vi "DisplayJson.vi"(11 "JSON String In":string="[{\"version\":\"1.0.0\",\"header\":{\"creationDate\":\"2022-06-03T00:00:00\",\"remarks\":\"\",\"serialNumber\":\"98172\",\"productNumber\":\"123021.1804\",\"productType\":\"PAA-9L\",\"pressureType\":2,\"productSeries\":\"9L\",\"compensatedTemperatureRange\":{\"min\":-10.0,\"max\":80.0,\"unit\":4},\"compensatedPressureRange\":{\"min\":0.0,\"max\":0.35,\"unit\":3},\"electricSupply\":{\"magnitude\":1.0,\"unit\":18},\"orderNumber\":9990266,\"orderPosition\":3,\"orderTargetDispatchDate\":\"2022-06-02T00:00:00+00:00\",\"customerName\":\"DemoData Inc.\",\"customerNumber\":12345678,\"customerOrderNumber\":\"Cust-9990266-123\",\"customerReferenceNumber\":\"\",\"customerProductT...") -> ()   [LabVIEW 2017] (continued)
nsatedPressureRange\":{\"min\":0.0,\"max\":0.35,\"unit\":3},\"electricSupply\":{\"magnitude\":1.0,\"unit\":18},\"parts\":{\"pressure\":{\"inputs\":[\"Sig\",\"R\"],\"output\":\"P\",\"description\":\"P = f(Sig,R)\",\"coefficients\":[[4.32580143572,-0.00440494166515,1.6640292116E-06,-2.811503068E-10,1.77714318789E-14],[-0.135698051026,0.000145399145759,-5.51829171562E-08,9.2954527005E-12,-5.87658681908E-16],[-0.000210397340774,2.63566870768E-07,-1.19781998432E-10,2.37289366107E-14,-1.74028064372E-18]]},\"temperature\":{\"inputs\":[\"R\",\"Sig\"],\"output\":\"T\",\"description\":\"T = f(R,Sig)\",\"coefficients\":[[-7912.16489659,3.11303262224,-0.10735561471],[7.82433050485,-0.00250618716574,0.000118515503682],[-0.00296929079857,7.28944709623E-07,-4.91144781497E-08],[5.10659036054E-07,-8.59548259995E-11,9.04763177647E-12],[-3.31476837963E-11,3.07780227507E-15,-6.24752257771E-16]]}}}}},\"measurements\":[{\"reference\":\"F_12300_XX_0000098765\",\"environmentTarget\":{\"pressure\":{\"magnitude\":0.03,\"unit\":3},\"temperature\":{\"magnitude\":-10.0,\"unit\":4}},\"environment\":{\"pressure\":{\"magnitude\":0.030005,\"unit\":3},\"temperature\":{\"magnitude\":-10.7286,\"unit\":4},\"supply\":{\"magnitude\":1.0,\"unit\":18}},\"raw\":{\"signal\":{\"magnitude\":15.068338109,\"unit\":22},\"bridgeResistance\":{\"magnitude\":3268.0076497,\"unit\":28}},\"compensated\":{\"mathematicalModels\":{\"MM0123\":{\"pressure\":{\"output\":{\"magnitude\":0.0300137,\"unit\":3},\"error\":{\"magnitude\":0.0024720218,\"unit\":7}},\"temperature\":{\"output\":{\"magnitude\":-10.8267,\"unit\":4},\"error\":{\"magnitude\":-0.098057362,\"unit\":4}}}}}},{\"reference\":\"F_12300_XX_0000098765\",\"environmentTarget\":{\"pressure\":{\"magnitude\":0.11,\"unit\":3},\"temperature\":{\"magnitude\":-10.0,\"unit\":4}},\"environment\":{\"pressure\":{\"magnitude\":0.109989,\"unit\":3},\"temperature\":{\"magnitude\":-10.7286,\"unit\":4},\"supply\":{\"magnitude\":1.0,\"unit\":18}},\"raw\":{\"signal\":{\"magnitude\":25.595891825,\"unit\":22},\"bridgeResistance\":{\"magnitude\":3264.0622557,\"unit\":28}},\"compensated\":{\"mathematicalModels\":{\"MM0123\":{\"pressure\":{\"output\":{\"magnitude\":0.10996,\"unit\":3},\"error\":{\"magnitude\":-0.0079711693,\"unit\":7}},\"temperature\":{\"output\":{\"magnitude\":-10.8338,\"unit\":4},\"error\":{\"magnitude\":-0.10516508,\"unit\":4}}}}}},{\"reference\":\"F_12300_XX_0000098765\",\"environmentTarget\":{\"pressure\":{\"magnitude\":0.19,\"unit\":3},\"temperature\":{\"magnitude\":-10.0,\"unit\":4}},\"environment\":{\"pressure\":{\"magnitude\":0.190009,\"unit\":3},\"temperature\":{\"magnitude\":-10.7286,\"unit\":4},\"supply\":{\"magnitude\":1.0,\"unit\":18}},\"raw\":{\"signal\":{\"magnitude\":36.103007271,\"unit\":22},\"bridgeResistance\":{\"magnitude\":3260.2938754,\"unit\":28}},\"compensated\":{\"mathematicalModels\":{\"MM0123\":{\"pressure\":{\"output\":{\"magnitude\":0.190015,\"unit\":3},\"error\":{\"magnitude\":0.001783636,\"unit\":7}},\"temperature\":{\"output\":{\"magnitude\":-10.8272,\"unit\":4},\"error\":{\"magnitude\":-0.098521286,\"unit\":4}}}}}},{\"reference\":\"F_12300_XX_0000098765\",\"environmentTarget\":{\"pressure\":{\"magnitude\":0.27,\"unit\":3},\"temperature\":{\"magnitude\":-10.0,\"unit\":4}},\"environment\":{\"pressure\":{\"magnitude\":0.270007,\"unit\":3},\"temperature\":{\"magnitude\":-10.7286,\"unit\":4},\"supply\":{\"magnitude\":1.0,\"unit\":18}},\"raw\":{\"signal\":{\"magnitude\":46.569581681,\"unit\":22},\"bridgeResistance\":{\"magnitude\":3256.5849623,\"unit\":28}},\"compensated\":{\"mathematicalModels\":{\"MM0123\":{\"pressure\":{\"output\":{\"magnitude\":0.270034,\"unit\":3},\"error\":{\"magnitude\":0.0075826501,\"unit\":7}},\"temperature\":{\"output\":{\"magnitude\":-10.8257,\"unit\":4},\"error\":{\"magnitude\":-0.097105964,\"unit\":4}}}}}},{\"reference\":\"F_12300_XX_0000098765\",\"environmentTarget\":{\"pressure\":{\"magnitude\":0.35,\"unit\":3},\"temperature\":{\"magnitude\":-10.0,\"unit\":4}},\"environment\":{\"pressure\":{\"magnitude\":0.350004,\"unit\":3},\"temperature\":{\"magnitude\":-10.7286,\"unit\":4},\"supply\":{\"magnitude\":1.0,\"unit\":18}},\"raw\":{\"signal\":{\"magnitude\":56.993492418,\"unit\":22},\"bridgeResistance\":{\"magnitude\":3252.9352126,\"unit\":28}},\"compensated\":{\"mathematicalModels\":{\"MM0123\":{\"pressure\":{\"output\":{\"magnitude\":0.35,\"unit\":3},\"error\":{\"magnitude\":-0.0012287617,\"unit\":7}},\"temperature\":{\"output\":{\"magnitude\":-10.83,\"unit\":4},\"error\":{\"magnitude\":-0.10133045,\"unit\":4}}}}}},{\"reference\":\"F_12300_XX_0000098765\",\"environmentTarget\":{\"pressure\":{\"magnitude\":0.03,\"unit\":3},\"temperature\":{\"magnitude\":0.0,\"unit\":4}},\"environment\":{\"pressure\":{\"magnitude\":0.0299941,\"unit\":3},\"temperature\":{\"magnitude\":-0.629962,\"unit\":4},\"supply\":{\"magnitude\":1.0,\"unit\":18}},\"raw\":{\"signal\":{\"magnitude\":15.503162041,\"unit\":22},\"bridgeResistance\":{\"magnitude\":3337.8630039,\"unit\":28}},\"compensated\":{\"mathematicalModels\":{\"MM0123\":{\"pressure\":{\"output\":{\"magnitude\":0.0300113,\"unit\":3},\"error\":{\"magnitude\":0.0049240687,\"unit\":7}},\"temperature\":{\"output\":{\"magnitude\":-0.740587,\"unit\":4},\"error\":{\"magnitude\":-0.1106252,\"unit\":4}}}}}},{\"reference\":\"F_12300_XX_0000098765\",\"environmentTarget\":{\"pressure\":{\"magnitude\":0.11,\"unit\":3},\"temperature\":{\"magnitude\":0.0,\"unit\":4}},\"environment\":{\"pressure\":{\"magnitude\":0.110002,\"unit\":3},\"temperature\":{\"magnitude\":-0.629962,\"unit\":4},\"supply\":{\"magnitude\":1.0,\"unit\":18}},\"raw\":{\"signal\":{\"magnitude\":26.002306136,\"unit\":22},\"bridgeResistance\":{\"magnitude\":3333.9686869,\"unit\":28}},\"compensated\":{\"mathematicalModels\":{\"MM0123\":{\"pressure\":{\"output\":{\"magnitude\":0.10998,\"unit\":3},\"error\":{\"magnitude\":-0.0063838503,\"unit\":7}},\"temperature\":{\"output\":{\"magnitude\":-0.740425,\"unit\":4},\"error\":{\"magnitude\":-0.11046359,\"unit\":4}}}}}},{\"reference\":\"F_12300_XX_0000098765\",\"environmentTarget\":{\"pressure\":{\"magnitude\":0.19,\"unit\":3},\"temperature\":{\"magnitude\":0.0,\"unit\":4}},\"environment\":{\"pressure\":{\"magnitude\":0.190006,\"unit\":3},\"temperature\":{\"magnitude\":-0.629962,\"unit\":4},\"supply\":{\"magnitude\":1.0,\"unit\":18}},\"raw\":{\"signal\":{\"magnitude\":36.476080101,\"unit\":22},\"bridgeResistance\":{\"magnitude\":3330.1476544,\"unit\":28}},\"compensated\":{\"mathematicalModels\":{\"MM0123\":{\"pressure\":{\"output\":{\"magnitude\":0.190009,\"unit\":3},\"error\":{\"magnitude\":0.0007371048,\"unit\":7}},\"temperature\":{\"output\":{\"magnitude\":-0.741023,\"unit\":4},\"error\":{\"magnitude\":-0.11206099,\"unit\":4}}}}}},{\"reference\":\"F_12300_XX_0000098765\",\"environmentTarget\":{\"pressure\":{\"magnitude\":0.27,\"unit\":3},\"temperature\":{\"magnitude\":0.0,\"unit\":4}},\"environment\":{\"pressure\":{\"magnitude\":0.269998,\"unit\":3},\"temperature\":{\"magnitude\":-0.629962,\"unit\":4},\"supply\":{\"magnitude\":1.0,\"unit\":18}},\"raw\":{\"signal\":{\"magnitude\":46.912344811,\"unit\":22},\"bridgeResistance\":{\"magnitude\":3326.3598207,\"unit\":28}},\"compensated\":{\"mathematicalModels\":{\"MM0123\":{\"pressure\":{\"output\":{\"magnitude\":0.270009,\"unit\":3},\"error\":{\"magnitude\":0.0030303754,\"unit\":7}},\"temperature\":{\"output\":{\"magnitude\":-0.748735,\"unit\":4},\"error\":{\"magnitude\":-0.11877286,\"unit\":4}}}}}},{\"reference\":\"F_12300_XX_0000098765\",\"environmentTarget\":{\"pressure\":{\"magnitude\":0.35,\"unit\":3},\"temperature\":{\"magnitude\":0.0,\"unit\":4}},\"environment\":{\"pressure\":{\"magnitude\":0.350003,\"unit\":3},\"temperature\":{\"magnitude\":-0.629962,\"unit\":4},\"supply\":{\"magnitude\":1.0,\"unit\":18}},\"raw\":{\"signal\":{\"magnitude\":57.311280041,\"unit\":22},\"bridgeResistance\":{\"magnitude\":3322.6985202,\"unit\":28}},\"compensated\":{\"mathematicalModels\":{\"MM0123\":{\"pressure\":{\"output\":{\"magnitude\":0.349978,\"unit\":3},\"error\":{\"magnitude\":-0.007067618,\"unit\":7}},\"temperature\":{\"output\":{\"magnitude\":-0.750753,\"unit\":4},\"error\":{\"magnitude\":-0.12079072,\"unit\":4}}}}}},{\"reference\":\"F_12300_XX_0000098765\",\"environmentTarget\":{\"pressure\":{\"magnitude\":0.03,\"unit\":3},\"temperature\":{\"magnitude\":20.0,\"unit\":4}},\"environment\":{\"pressure\":{\"magnitude\":0.0299999,\"unit\":3},\"temperature\":{\"magnitude\":19.5509,\"unit\":4},\"supply\":{\"magnitude\":1.0,\"unit\":18}},\"raw\":{\"signal\":{\"magnitude\":16.409278781,\"unit\":22},\"bridgeResistance\":{\"magnitude\":3494.5350045,\"unit\":28}},\"compensated\":{\"mathematicalModels\":{\"MM0123\":{\"pressure\":{\"output\":{\"magnitude\":0.0300059,\"unit\":3},\"error\":{\"magnitude\":0.0017026825,\"unit\":7}},\"temperature\":{\"output\":{\"magnitude\":19.5499,\"unit\":4},\"error\":{\"magnitude\":-0.0009297112,\"unit\":4}}}}}},{\"reference\":\"F_12300_XX_0000098765\",\"environmentTarget\":{\"pressure\":{\"magnitude\":0.11,\"unit\":3},\"temperature\":{\"magnitude\":20.0,\"unit\":4}},\"environment\":{\"pressure\":{\"magnitude\":0.109998,\"unit\":3},\"temperature\":{\"magnitude\":19.5509,\"unit\":4},\"supply\":{\"magnitude\":1.0,\"unit\":18}},\"raw\":{\"signal\":{\"magnitude\":26.89717523,\"unit\":22},\"bridgeResistance\":{\"magnitude\":3490.6076187,\"unit\":28}},\"compensated\":{\"mathematicalModels\":{\"MM0123\":{\"pressure\":{\"output\":{\"magnitude\":0.109972,\"unit\":3},\"error\":{\"magnitude\":-0.0073489568,\"unit\":7}},\"temperature\":{\"output\":{\"magnitude\":19.5448,\"unit\":4},\"error\":{\"magnitude\":-0.0060927679,\"unit\":4}}}}}},{\"reference\":\"F_12300_XX_0000098765\",\"environmentTarget\":{\"pressure\":{\"magnitude\":0.19,\"unit\":3},\"temperature\":{\"magnitude\":20.0,\"unit\":4}},\"environment\":{\"pressure\":{\"magnitude\":0.189997,\"unit\":3},\"temperature\":{\"magnitude\":19.5509,\"unit\":4},\"supply\":{\"magnitude\":1.0,\"unit\":18}},\"raw\":{\"signal\":{\"magnitude\":37.363996162,\"unit\":22},\"bridgeResistance\":{\"magnitude\":3486.7813876,\"unit\":28}},\"compensated\":{\"mathematicalModels\":{\"MM0123\":{\"pressure\":{\"output\":{\"magnitude\":0.190001,\"unit\":3},\"error\":{\"magnitude\":0.0011381596,\"unit\":7}},\"temperature\":{\"output\":{\"magnitude\":19.5437,\"unit\":4},\"error\":{\"magnitude\":-0.0071879925,\"unit\":4}}}}}},{\"reference\":\"F_12300_XX_0000098765\",\"environmentTarget\":{\"pressure\":{\"magnitude\":0.27,\"unit\":3},\"temperature\":{\"magnitude\":20.0,\"unit\":4}},\"environment\":{\"pressure\":{\"magnitude\":0.269992,\"unit\":3},\"temperature\":{\"magnitude\":19.5509,\"unit\":4},\"supply\":{\"magnitude\":1.0,\"unit\":18}},\"raw\":{\"signal\":{\"magnitude\":47.800155632,\"unit\":22},\"bridgeResistance\":{\"magnitude\":3483.0010425,\"unit\":28}},\"compensated\":{\"mathematicalModels\":{\"MM0123\":{\"pressure\":{\"output\":{\"magnitude\":0.270022,\"unit\":3},\"error\":{\"magnitude\":0.008607717,\"unit\":7}},\"temperature\":{\"output\":{\"magnitude\":19.5395,\"unit\":4},\"error\":{\"magnitude\":-0.011423775,\"unit\":4}}}}}},{\"reference\":\"F_12300_XX_0000098765\",\"environmentTarget\":{\"pressure\":{\"magnitude\":0.35,\"unit\":3},\"temperature\":{\"magnitude\":20.0,\"unit\":4}},\"environment\":{\"pressure\":{\"magnitude\":0.350005,\"unit\":3},\"temperature\":{\"magnitude\":19.5509,\"unit\":4},\"supply\":{\"magnitude\":1.0,\"unit\":18}},\"raw\":{\"signal\":{\"magnitude\":58.202570119,\"unit\":22},\"bridgeResistance\":{\"magnitude\":3479.3453591,\"unit\":28}},\"compensated\":{\"mathematicalModels\":{\"MM0123\":{\"pressure\":{\"output\":{\"magnitude\":0.350009,\"unit\":3},\"error\":{\"magnitude\":0.0010923873,\"unit\":7}},\"temperature\":{\"output\":{\"magnitude\":19.5414,\"unit\":4},\"error\":{\"magnitude\":-0.009468969,\"unit\":4}}}}}},{\"reference\":\"F_12300_XX_0000098765\",\"environmentTarget\":{\"pressure\":{\"magnitude\":0.03,\"unit\":3},\"temperature\":{\"magnitude\":40.0,\"unit\":4}},\"environment\":{\"pressure\":{\"magnitude\":0.0299981,\"unit\":3},\"temperature\":{\"magnitude\":39.7284,\"unit\":4},\"supply\":{\"magnitude\":1.0,\"unit\":18}},\"raw\":{\"signal\":{\"magnitude\":17.383077086,\"unit\":22},\"bridgeResistance\":{\"magnitude\":3670.0301141,\"unit\":28}},\"compensated\":{\"mathematicalModels\":{\"MM0123\":{\"pressure\":{\"output\":{\"magnitude\":0.0300152,\"unit\":3},\"error\":{\"magnitude\":0.0048902957,\"unit\":7}},\"temperature\":{\"output\":{\"magnitude\":39.719,\"unit\":4},\"error\":{\"magnitude\":-0.0094604345,\"unit\":4}}}}}},{\"reference\":\"F_12300_XX_0000098765\",\"environmentTarget\":{\"pressure\":{\"magnitude\":0.11,\"unit\":3},\"temperature\":{\"magnitude\":40.0,\"unit\":4}},\"environment\":{\"pressure\":{\"magnitude\":0.109992,\"unit\":3},\"temperature\":{\"magnitude\":39.7284,\"unit\":4},\"supply\":{\"magnitude\":1.0,\"unit\":18}},\"raw\":{\"signal\":{\"magnitude\":27.915913124,\"unit\":22},\"bridgeResistance\":{\"magnitude\":3666.1287959,\"unit\":28}},\"compensated\":{\"mathematicalModels\":{\"MM0123\":{\"pressure\":{\"output\":{\"magnitude\":0.109964,\"unit\":3},\"error\":{\"magnitude\":-0.0079924079,\"unit\":7}},\"temperature\":{\"output\":{\"magnitude\":39.718,\"unit\":4},\"error\":{\"magnitude\":-0.010393948,\"unit\":4}}}}}},{\"reference\":\"F_12300_XX_0000098765\",\"environmentTarget\":{\"pressure\":{\"magnitude\":0.19,\"unit\":3},\"temperature\":{\"magnitude\":40.0,\"unit\":4}},\"environment\":{\"pressure\":{\"magnitude\":0.190002,\"unit\":3},\"temperature\":{\"magnitude\":39.7284,\"unit\":4},\"supply\":{\"magnitude\":1.0,\"unit\":18}},\"raw\":{\"signal\":{\"magnitude\":38.435222706,\"unit\":22},\"bridgeResistance\":{\"magnitude\":3662.2737602,\"unit\":28}},\"compensated\":{\"mathematicalModels\":{\"MM0123\":{\"pressure\":{\"output\":{\"magnitude\":0.190008,\"unit\":3},\"error\":{\"magnitude\":0.0016626825,\"unit\":7}},\"temperature\":{\"output\":{\"magnitude\":39.7163,\"unit\":4},\"error\":{\"magnitude\":-0.012099664,\"unit\":4}}}}}},{\"reference\":\"F_12300_XX_0000098765\",\"environmentTarget\":{\"pressure\":{\"magnitude\":0.27,\"unit\":3},\"temperature\":{\"magnitude\":40.0,\"unit\":4}},\"environment\":{\"pressure\":{\"magnitude\":0.270007,\"unit\":3},\"temperature\":{\"magnitude\":39.7284,\"unit\":4},\"supply\":{\"magnitude\":1.0,\"unit\":18}},\"raw\":{\"signal\":{\"magnitude\":48.924402683,\"unit\":22},\"bridgeResistance\":{\"magnitude\":3658.4937993,\"unit\":28}},\"compensated\":{\"mathematicalModels\":{\"MM0123\":{\"pressure\":{\"output\":{\"magnitude\":0.27002,\"unit\":3},\"error\":{\"magnitude\":0.0035956822,\"unit\":7}},\"temperature\":{\"output\":{\"magnitude\":39.7162,\"unit\":4},\"error\":{\"magnitude\":-0.012215598,\"unit\":4}}}}}},{\"reference\":\"F_12300_XX_0000098765\",\"environmentTarget\":{\"pressure\":{\"magnitude\":0.35,\"unit\":3},\"temperature\":{\"magnitude\":40.0,\"unit\":4}},\"environment\":{\"pressure\":{\"magnitude\":0.349997,\"unit\":3},\"temperature\":{\"magnitude\":39.7284,\"unit\":4},\"supply\":{\"magnitude\":1.0,\"unit\":18}},\"raw\":{\"signal\":{\"magnitude\":59.380068238,\"unit\":22},\"bridgeResistance\":{\"magnitude\":3654.7298992,\"unit\":28}},\"compensated\":{\"mathematicalModels\":{\"MM0123\":{\"pressure\":{\"output\":{\"magnitude\":0.349976,\"unit\":3},\"error\":{\"magnitude\":-0.0058753456,\"unit\":7}},\"temperature\":{\"output\":{\"magnitude\":39.711,\"unit\":4},\"error\":{\"magnitude\":-0.017436603,\"unit\":4}}}}}},{\"reference\":\"F_12300_XX_0000098765\",\"environmentTarget\":{\"pressure\":{\"magnitude\":0.03,\"unit\":3},\"temperature\":{\"magnitude\":60.0,\"unit\":4}},\"environment\":{\"pressure\":{\"magnitude\":0.0300107,\"unit\":3},\"temperature\":{\"magnitude\":59.8651,\"unit\":4},\"supply\":{\"magnitude\":1.0,\"unit\":18}},\"raw\":{\"signal\":{\"magnitude\":18.466369717,\"unit\":22},\"bridgeResistance\":{\"magnitude\":3861.7940032,\"unit\":28}},\"compensated\":{\"mathematicalModels\":{\"MM0123\":{\"pressure\":{\"output\":{\"magnitude\":0.030024,\"unit\":3},\"error\":{\"magnitude\":0.0037926278,\"unit\":7}},\"temperature\":{\"output\":{\"magnitude\":59.9257,\"unit\":4},\"error\":{\"magnitude\":0.060552346,\"unit\":4}}}}}},{\"reference\":\"F_12300_XX_0000098765\",\"environmentTarget\":{\"pressure\":{\"magnitude\":0.11,\"unit\":3},\"temperature\":{\"magnitude\":60.0,\"unit\":4}},\"environment\":{\"pressure\":{\"magnitude\":0.110004,\"unit\":3},\"temperature\":{\"magnitude\":59.8651,\"unit\":4},\"supply\":{\"magnitude\":1.0,\"unit\":18}},\"raw\":{\"signal\":{\"magnitude\":29.082015037,\"unit\":22},\"bridgeResistance\":{\"magnitude\":3857.8526834,\"unit\":28}},\"compensated\":{\"mathematicalModels\":{\"MM0123\":{\"pressure\":{\"output\":{\"magnitude\":0.109974,\"unit\":3},\"error\":{\"magnitude\":-0.0085022978,\"unit\":7}},\"temperature\":{\"output\":{\"magnitude\":59.9272,\"unit\":4},\"error\":{\"magnitude\":0.0620527,\"unit\":4}}}}}},{\"reference\":\"F_12300_XX_0000098765\",\"environmentTarget\":{\"pressure\":{\"magnitude\":0.19,\"unit\":3},\"temperature\":{\"magnitude\":60.0,\"unit\":4}},\"environment\":{\"pressure\":{\"magnitude\":0.189991,\"unit\":3},\"temperature\":{\"magnitude\":59.8651,\"unit\":4},\"supply\":{\"magnitude\":1.0,\"unit\":18}},\"raw\":{\"signal\":{\"magnitude\":39.684819017,\"unit\":22},\"bridgeResistance\":{\"magnitude\":3853.9571362,\"unit\":28}},\"compensated\":{\"mathematicalModels\":{\"MM0123\":{\"pressure\":{\"output\":{\"magnitude\":0.189998,\"unit\":3},\"error\":{\"magnitude\":0.0019648268,\"unit\":7}},\"temperature\":{\"output\":{\"magnitude\":59.93,\"unit\":4},\"error\":{\"magnitude\":0.064823338,\"unit\":4}}}}}},{\"reference\":\"F_12300_XX_0000098765\",\"environmentTarget\":{\"pressure\":{\"magnitude\":0.27,\"unit\":3},\"temperature\":{\"magnitude\":60.0,\"unit\":4}},\"environment\":{\"pressure\":{\"magnitude\":0.270005,\"unit\":3},\"temperature\":{\"magnitude\":59.8651,\"unit\":4},\"supply\":{\"magnitude\":1.0,\"unit\":18}},\"raw\":{\"signal\":{\"magnitude\":50.265641319,\"unit\":22},\"bridgeResistance\":{\"magnitude\":3850.0680121,\"unit\":28}},\"compensated\":{\"mathematicalModels\":{\"MM0123\":{\"pressure\":{\"output\":{\"magnitude\":0.270029,\"unit\":3},\"error\":{\"magnitude\":0.006864249,\"unit\":7}},\"temperature\":{\"output\":{\"magnitude\":59.9296,\"unit\":4},\"error\":{\"magnitude\":0.064421463,\"unit\":4}}}}}},{\"reference\":\"F_12300_XX_0000098765\",\"environmentTarget\":{\"pressure\":{\"magnitude\":0.35,\"unit\":3},\"temperature\":{\"magnitude\":60.0,\"unit\":4}},\"environment\":{\"pressure\":{\"magnitude\":0.349992,\"unit\":3},\"temperature\":{\"magnitude\":59.8651,\"unit\":4},\"supply\":{\"magnitude\":1.0,\"unit\":18}},\"raw\":{\"signal\":{\"magnitude\":60.813927022,\"unit\":22},\"bridgeResistance\":{\"magnitude\":3846.2738985,\"unit\":28}},\"compensated\":{\"mathematicalModels\":{\"MM0123\":{\"pressure\":{\"output\":{\"magnitude\":0.349984,\"unit\":3},\"error\":{\"magnitude\":-0.0023994201,\"unit\":7}},\"temperature\":{\"output\":{\"magnitude\":59.9345,\"unit\":4},\"error\":{\"magnitude\":0.06933577,\"unit\":4}}}}}},{\"reference\":\"F_12300_XX_0000098765\",\"environmentTarget\":{\"pressure\":{\"magnitude\":0.03,\"unit\":3},\"temperature\":{\"magnitude\":80.0,\"unit\":4}},\"environment\":{\"pressure\":{\"magnitude\":0.0299895,\"unit\":3},\"temperature\":{\"magnitude\":79.9513,\"unit\":4},\"supply\":{\"magnitude\":1.0,\"unit\":18}},\"raw\":{\"signal\":{\"magnitude\":19.701808057,\"unit\":22},\"bridgeResistance\":{\"magnitude\":4068.7761297,\"unit\":28}},\"compensated\":{\"mathematicalModels\":{\"MM0123\":{\"pressure\":{\"output\":{\"magnitude\":0.0300054,\"unit\":3},\"error\":{\"magnitude\":0.0048280872,\"unit\":7}},\"temperature\":{\"output\":{\"magnitude\":80.0425,\"unit\":4},\"error\":{\"magnitude\":0.091164426,\"unit\":4}}}}}},{\"reference\":\"F_12300_XX_0000098765\",\"environmentTarget\":{\"pressure\":{\"magnitude\":0.11,\"unit\":3},\"temperature\":{\"magnitude\":80.0,\"unit\":4}},\"environment\":{\"pressure\":{\"magnitude\":0.110002,\"unit\":3},\"temperature\":{\"magnitude\":79.9513,\"unit\":4},\"supply\":{\"magnitude\":1.0,\"unit\":18}},\"raw\":{\"signal\":{\"magnitude\":30.424082899,\"unit\":22},\"bridgeResistance\":{\"magnitude\":4064.7419553,\"unit\":28}},\"compensated\":{\"mathematicalModels\":{\"MM0123\":{\"pressure\":{\"output\":{\"magnitude\":0.109957,\"unit\":3},\"error\":{\"magnitude\":-0.012974161,\"unit\":7}},\"temperature\":{\"output\":{\"magnitude\":80.0438,\"unit\":4},\"error\":{\"magnitude\":0.092419126,\"unit\":4}}}}}},{\"reference\":\"F_12300_XX_0000098765\",\"environmentTarget\":{\"pressure\":{\"magnitude\":0.19,\"unit\":3},\"temperature\":{\"magnitude\":80.0,\"unit\":4}},\"environment\":{\"pressure\":{\"magnitude\":0.190011,\"unit\":3},\"temperature\":{\"magnitude\":79.9513,\"unit\":4},\"supply\":{\"magnitude\":1.0,\"unit\":18}},\"raw\":{\"signal\":{\"magnitude\":41.144759975,\"unit\":22},\"bridgeResistance\":{\"magnitude\":4060.8034636,\"unit\":28}},\"compensated\":{\"mathematicalModels\":{\"MM0123\":{\"pressure\":{\"output\":{\"magnitude\":0.19002,\"unit\":3},\"error\":{\"magnitude\":0.0025314902,\"unit\":7}},\"temperature\":{\"output\":{\"magnitude\":80.0504,\"unit\":4},\"error\":{\"magnitude\":0.099021935,\"unit\":4}}}}}},{\"reference\":\"F_12300_XX_0000098765\",\"environmentTarget\":{\"pressure\":{\"magnitude\":0.27,\"unit\":3},\"temperature\":{\"magnitude\":80.0,\"unit\":4}},\"environment\":{\"pressure\":{\"magnitude\":0.270008,\"unit\":3},\"temperature\":{\"magnitude\":79.9513,\"unit\":4},\"supply\":{\"magnitude\":1.0,\"unit\":18}},\"raw\":{\"signal\":{\"magnitude\":51.842284556,\"unit\":22},\"bridgeResistance\":{\"magnitude\":4056.9227234,\"unit\":28}},\"compensated\":{\"mathematicalModels\":{\"MM0123\":{\"pressure\":{\"output\":{\"magnitude\":0.270039,\"unit\":3},\"error\":{\"magnitude\":0.0089760869,\"unit\":7}},\"temperature\":{\"output\":{\"magnitude\":80.0584,\"unit\":4},\"error\":{\"magnitude\":0.10704536,\"unit\":4}}}}}},{\"reference\":\"F_12300_XX_0000098765\",\"environmentTarget\":{\"pressure\":{\"magnitude\":0.35,\"unit\":3},\"temperature\":{\"magnitude\":80.0,\"unit\":4}},\"environment\":{\"pressure\":{\"magnitude\":0.349999,\"unit\":3},\"temperature\":{\"magnitude\":79.9513,\"unit\":4},\"supply\":{\"magnitude\":1.0,\"unit\":18}},\"raw\":{\"signal\":{\"magnitude\":62.51145925,\"unit\":22},\"bridgeResistance\":{\"magnitude\":4053.0189189,\"unit\":28}},\"compensated\":{\"mathematicalModels\":{\"MM0123\":{\"pressure\":{\"output\":{\"magnitude\":0.349983,\"unit\":3},\"error\":{\"magnitude\":-0.0046507517,\"unit\":7}},\"temperature\":{\"output\":{\"magnitude\":80.0605,\"unit\":4},\"error\":{\"magnitude\":0.10915966,\"unit\":4}}}}}}]},{\"version\":\"1.0.0\",\"header\":{\"creationDate\":\"2022-06-03T00:00:00\",\"remarks\":\"\",\"serialNumber\":\"98037\",\"productNumber\":\"123021.1804\",\"productType\":\"PAA-9L\",\"pressureType\":2,\"productSeries\":\"9L\",\"compensatedTemperatureRange\":{\"min\":-10.0,\"max\":80.0,\"unit\":4},\"compensatedPressureRange\":{\"min\":0.0,\"max\":0.35,\"unit\":3},\"electricSupply\":{\"magnitude\":1.0,\"unit\":18},\"orderNumber\":9990266,\"orderPosition\":3,\"orderTargetDispatchDate\":\"2022-06-02T00:00:00+00:00\",\"customerName\":\"DemoData Inc.\",\"customerNumber\":12345678,\"customerOrderNumber\":\"Cust-9990266-123\",\"customerReferenceNumber\":\"\",\"customerProductType\":\"123021-1804 Rev.AA\"},\"compensationMethods\":{\"mathematicalModels\":{\"MM0123\":{\"modelType\":\"MM0123\",\"productNumber\":\"000000.0000\",\"compensatedTemperatureRange\":{\"min\":-10.0,\"max\":80.0,\"unit\":4},\"compensatedPressureRange\":{\"min\":0.0,\"max\":0.35,\"unit\":3},\"electricSupply\":{\"magnitude\":1.0,\"unit\":18},\"parts\":{\"pressure\":{\"inputs\":[\"Sig\",\"R\"],\"output\":\"P\",\"description\":\"P = f(Sig,R)\",\"coefficients\":[[4.00585239409,-0.00407660303892,1.54001645633E-06,-2.60531242099E-10,1.65145046643E-14],[-0.145780031109,0.000156267662266,-5.97442761532E-08,1.01497169125E-11,-6.47716190447E-16],[8.28923900558E-05,-6.47619287081E-08,1.77853613631E-11,-1.84069073647E-15,3.86832105217E-20]]},\"temperature\":{\"inputs\":[\"R\",\"Sig\"],\"output\":\"T\",\"description\":\"T = f(R,Sig)\",\"coefficients\":[[-8335.86951546,13.3053464608,-0.163740878138],[8.16522510022,-0.0132555975812,0.000175507767272],[-0.00306367704035,4.97458478986E-06,-7.05116702538E-08],[5.20224914659E-07,-8.301971996E-10,1.2579207023E-11],[-3.33202938189E-11,5.19268406667E-14,-8.40569563715E-16]]}}}}},\"measurements\":[{\"reference\":\"F_12300_XX_0000098765\",\"environmentTarget\":{\"pressure\":{\"magnitude\":0.03,\"unit\":3},\"temperature\":{\"magnitude\":-10.0,\"unit\":4}},\"environment\":{\"pressure\":{\"magnitude\":0.0300034,\"unit\":3},\"temperature\":{\"magnitude\":-10.7286,\"unit\":4},\"supply\":{\"magnitude\":1.0,\"unit\":18}},\"raw\":{\"signal\":{\"magnitude\":15.181513313,\"unit\":22},\"bridgeResistance\":{\"magnitude\":3290.5264503,\"unit\":28}},\"compensated\":{\"mathematicalModels\":{\"MM0123\":{\"pressure\":{\"output\":{\"magnitude\":0.030015,\"unit\":3},\"error\":{\"magnitude\":0.0033076453,\"unit\":7}},\"temperature\":{\"output\":{\"magnitude\":-10.8254,\"unit\":4},\"error\":{\"magnitude\":-0.096746731,\"unit\":4}}}}}},{\"reference\":\"F_12300_XX_0000098765\",\"environmentTarget\":{\"pressure\":{\"magnitude\":0.11,\"unit\":3},\"temperature\":{\"magnitude\":-10.0,\"unit\":4}},\"environment\":{\"pressure\":{\"magnitude\":0.110008,\"unit\":3},\"temperature\":{\"magnitude\":-10.7286,\"unit\":4},\"supply\":{\"magnitude\":1.0,\"unit\":18}},\"raw\":{\"signal\":{\"magnitude\":26.150631828,\"unit\":22},\"bridgeResistance\":{\"magnitude\":3286.3808984,\"unit\":28}},\"compensated\":{\"mathematicalModels\":{\"MM0123\":{\"pressure\":{\"output\":{\"magnitude\":0.109977,\"unit\":3},\"error\":{\"magnitude\":-0.0089115074,\"unit\":7}},\"temperature\":{\"output\":{\"magnitude\":-10.8321,\"unit\":4},\"error\":{\"magnitude\":-0.10347546,\"unit\":4}}}}}},{\"reference\":\"F_12300_XX_0000098765\",\"environmentTarget\":{\"pressure\":{\"magnitude\":0.19,\"unit\":3},\"temperature\":{\"magnitude\":-10.0,\"unit\":4}},\"environment\":{\"pressure\":{\"magnitude\":0.189999,\"unit\":3},\"temperature\":{\"magnitude\":-10.7286,\"unit\":4},\"supply\":{\"magnitude\":1.0,\"unit\":18}},\"raw\":{\"signal\":{\"magnitude\":37.090941156,\"unit\":22},\"bridgeResistance\":{\"magnitude\":3282.4084117,\"unit\":28}},\"compensated\":{\"mathematicalModels\":{\"MM0123\":{\"pressure\":{\"output\":{\"magnitude\":0.190006,\"unit\":3},\"error\":{\"magnitude\":0.002137079,\"unit\":7}},\"temperature\":{\"output\":{\"magnitude\":-10.827,\"unit\":4},\"error\":{\"magnitude\":-0.098408051,\"unit\":4}}}}}},{\"reference\":\"F_12300_XX_0000098765\",\"environmentTarget\":{\"pressure\":{\"magnitude\":0.27,\"unit\":3},\"temperature\":{\"magnitude\":-10.0,\"unit\":4}},\"environment\":{\"pressure\":{\"magnitude\":0.270006,\"unit\":3},\"temperature\":{\"magnitude\":-10.7286,\"unit\":4},\"supply\":{\"magnitude\":1.0,\"unit\":18}},\"raw\":{\"signal\":{\"magnitude\":47.991790468,\"unit\":22},\"bridgeResistance\":{\"magnitude\":3278.5082444,\"unit\":28}},\"compensated\":{\"mathematicalModels\":{\"MM0123\":{\"pressure\":{\"output\":{\"magnitude\":0.270033,\"unit\":3},\"error\":{\"magnitude\":0.0076839462,\"unit\":7}},\"temperature\":{\"output\":{\"magnitude\":-10.8267,\"unit\":4},\"error\":{\"magnitude\":-0.098045997,\"unit\":4}}}}}},{\"reference\":\"F_12300_XX_0000098765\",\"environmentTarget\":{\"pressure\":{\"magnitude\":0.35,\"unit\":3},\"temperature\":{\"magnitude\":-10.0,\"unit\":4}},\"environment\":{\"pressure\":{\"magnitude\":0.350006,\"unit\":3},\"temperature\":{\"magnitude\":-10.7286,\"unit\":4},\"supply\":{\"magnitude\":1.0,\"unit\":18}},\"raw\":{\"signal\":{\"magnitude\":58.845416791,\"unit\":22},\"bridgeResistance\":{\"magnitude\":3274.693759,\"unit\":28}},\"compensated\":{\"mathematicalModels\":{\"MM0123\":{\"pressure\":{\"output\":{\"magnitude\":0.35,\"unit\":3},\"error\":{\"magnitude\":-0.0016762531,\"unit\":7}},\"temperature\":{\"output\":{\"magnitude\":-10.83,\"unit\":4},\"error\":{\"magnitude\":-0.10140449,\"unit\":4}}}}}},{\"reference\":\"F_12300_XX_0000098765\",\"environmentTarget\":{\"pressure\":{\"magnitude\":0.03,\"unit\":3},\"temperature\":{\"magnitude\":0.0,\"unit\":4}},\"environment\":{\"pressure\":{\"magnitude\":0.0300026,\"unit\":3},\"temperature\":{\"magnitude\":-0.629962,\"unit\":4},\"supply\":{\"magnitude\":1.0,\"unit\":18}},\"raw\":{\"signal\":{\"magnitude\":15.591789572,\"unit\":22},\"bridgeResistance\":{\"magnitude\":3359.683895,\"unit\":28}},\"compensated\":{\"mathematicalModels\":{\"MM0123\":{\"pressure\":{\"output\":{\"magnitude\":0.0300183,\"unit\":3},\"error\":{\"magnitude\":0.0044866792,\"unit\":7}},\"temperature\":{\"output\":{\"magnitude\":-0.735029,\"unit\":4},\"error\":{\"magnitude\":-0.10506732,\"unit\":4}}}}}},{\"reference\":\"F_12300_XX_0000098765\",\"environmentTarget\":{\"pressure\":{\"magnitude\":0.11,\"unit\":3},\"temperature\":{\"magnitude\":0.0,\"unit\":4}},\"environment\":{\"pressure\":{\"magnitude\":0.110005,\"unit\":3},\"temperature\":{\"magnitude\":-0.629962,\"unit\":4},\"supply\":{\"magnitude\":1.0,\"unit\":18}},\"raw\":{\"signal\":{\"magnitude\":26.529939949,\"unit\":22},\"bridgeResistance\":{\"magnitude\":3355.6101064,\"unit\":28}},\"compensated\":{\"mathematicalModels\":{\"MM0123\":{\"pressure\":{\"output\":{\"magnitude\":0.10998,\"unit\":3},\"error\":{\"magnitude\":-0.0072470297,\"unit\":7}},\"temperature\":{\"output\":{\"magnitude\":-0.73609,\"unit\":4},\"error\":{\"magnitude\":-0.10612818,\"unit\":4}}}}}},{\"reference\":\"F_12300_XX_0000098765\",\"environmentTarget\":{\"pressure\":{\"magnitude\":0.19,\"unit\":3},\"temperature\":{\"magnitude\":0.0,\"unit\":4}},\"environment\":{\"pressure\":{\"magnitude\":0.190006,\"unit\":3},\"temperature\":{\"magnitude\":-0.629962,\"unit\":4},\"supply\":{\"magnitude\":1.0,\"unit\":18}},\"raw\":{\"signal\":{\"magnitude\":37.440497654,\"unit\":22},\"bridgeResistance\":{\"magnitude\":3351.6309573,\"unit\":28}},\"compensated\":{\"mathematicalModels\":{\"MM0123\":{\"pressure\":{\"output\":{\"magnitude\":0.190005,\"unit\":3},\"error\":{\"magnitude\":-0.00031554597,\"unit\":7}},\"temperature\":{\"output\":{\"magnitude\":-0.734964,\"unit\":4},\"error\":{\"magnitude\":-0.10500255,\"unit\":4}}}}}},{\"reference\":\"F_12300_XX_0000098765\",\"environmentTarget\":{\"pressure\":{\"magnitude\":0.27,\"unit\":3},\"temperature\":{\"magnitude\":0.0,\"unit\":4}},\"environment\":{\"pressure\":{\"magnitude\":0.269997,\"unit\":3},\"temperature\":{\"magnitude\":-0.629962,\"unit\":4},\"supply\":{\"magnitude\":1.0,\"unit\":18}},\"raw\":{\"signal\":{\"magnitude\":48.311960193,\"unit\":22},\"bridgeResistance\":{\"magnitude\":3347.6921213,\"unit\":28}},\"compensated\":{\"mathematicalModels\":{\"MM0123\":{\"pressure\":{\"output\":{\"magnitude\":0.270014,\"unit\":3},\"error\":{\"magnitude\":0.0047220373,\"unit\":7}},\"temperature\":{\"output\":{\"magnitude\":-0.740207,\"unit\":4},\"error\":{\"magnitude\":-0.11024518,\"unit\":4}}}}}},{\"reference\":\"F_12300_XX_0000098765\",\"environmentTarget\":{\"pressure\":{\"magnitude\":0.35,\"unit\":3},\"temperature\":{\"magnitude\":0.0,\"unit\":4}},\"environment\":{\"pressure\":{\"magnitude\":0.350002,\"unit\":3},\"temperature\":{\"magnitude\":-0.629962,\"unit\":4},\"supply\":{\"magnitude\":1.0,\"unit\":18}},\"raw\":{\"signal\":{\"magnitude\":59.140724357,\"unit\":22},\"bridgeResistance\":{\"magnitude\":3343.8543557,\"unit\":28}},\"compensated\":{\"mathematicalModels\":{\"MM0123\":{\"pressure\":{\"output\":{\"magnitude\":0.349978,\"unit\":3},\"error\":{\"magnitude\":-0.0069461893,\"unit\":7}},\"temperature\":{\"output\":{\"magnitude\":-0.743843,\"unit\":4},\"error\":{\"magnitude\":-0.11389123,\"unit\":4}}}}}},{\"reference\":\"F_12300_XX_0000098765\",\"environmentTarget\":{\"pressure\":{\"magnitude\":0.03,\"unit\":3},\"temperature\":{\"magnitude\":20.0,\"unit\":4}},\"environment\":{\"pressure\":{\"magnitude\":0.0300076,\"unit\":3},\"temperature\":{\"magnitude\":19.5509,\"unit\":4},\"supply\":{\"magnitude\":1.0,\"unit\":18}},\"raw\":{\"signal\":{\"magnitude\":16.457385982,\"unit\":22},\"bridgeResistance\":{\"magnitude\":3515.5266428,\"unit\":28}},\"compensated\":{\"mathematicalModels\":{\"MM0123\":{\"pressure\":{\"output\":{\"magnitude\":0.0300186,\"unit\":3},\"error\":{\"magnitude\":0.0031460311,\"unit\":7}},\"temperature\":{\"output\":{\"magnitude\":19.5484,\"unit\":4},\"error\":{\"magnitude\":-0.002525709,\"unit\":4}}}}}},{\"reference\":\"F_12300_XX_0000098765\",\"environmentTarget\":{\"pressure\":{\"magnitude\":0.11,\"unit\":3},\"temperature\":{\"magnitude\":20.0,\"unit\":4}},\"environment\":{\"pressure\":{\"magnitude\":0.110002,\"unit\":3},\"temperature\":{\"magnitude\":19.5509,\"unit\":4},\"supply\":{\"magnitude\":1.0,\"unit\":18}},\"raw\":{\"signal\":{\"magnitude\":27.38391793,\"unit\":22},\"bridgeResistance\":{\"magnitude\":3511.4167623,\"unit\":28}},\"compensated\":{\"mathematicalModels\":{\"MM0123\":{\"pressure\":{\"output\":{\"magnitude\":0.109973,\"unit\":3},\"error\":{\"magnitude\":-0.0083140051,\"unit\":7}},\"temperature\":{\"output\":{\"magnitude\":19.5411,\"unit\":4},\"error\":{\"magnitude\":-0.0097790006,\"unit\":4}}}}}},{\"reference\":\"F_12300_XX_0000098765\",\"environmentTarget\":{\"pressure\":{\"magnitude\":0.19,\"unit\":3},\"temperature\":{\"magnitude\":20.0,\"unit\":4}},\"environment\":{\"pressure\":{\"magnitude\":0.189993,\"unit\":3},\"temperature\":{\"magnitude\":19.5509,\"unit\":4},\"supply\":{\"magnitude\":1.0,\"unit\":18}},\"raw\":{\"signal\":{\"magnitude\":38.289297975,\"unit\":22},\"bridgeResistance\":{\"magnitude\":3507.4197814,\"unit\":28}},\"compensated\":{\"mathematicalModels\":{\"MM0123\":{\"pressure\":{\"output\":{\"magnitude\":0.190001,\"unit\":3},\"error\":{\"magnitude\":0.0021955479,\"unit\":7}},\"temperature\":{\"output\":{\"magnitude\":19.5395,\"unit\":4},\"error\":{\"magnitude\":-0.011378321,\"unit\":4}}}}}},{\"reference\":\"F_12300_XX_0000098765\",\"environmentTarget\":{\"pressure\":{\"magnitude\":0.27,\"unit\":3},\"temperature\":{\"magnitude\":20.0,\"unit\":4}},\"environment\":{\"pressure\":{\"magnitude\":0.269993,\"unit\":3},\"temperature\":{\"magnitude\":19.5509,\"unit\":4},\"supply\":{\"magnitude\":1.0,\"unit\":18}},\"raw\":{\"signal\":{\"magnitude\":49.159269078,\"unit\":22},\"bridgeResistance\":{\"magnitude\":3503.466789,\"unit\":28}},\"compensated\":{\"mathematicalModels\":{\"MM0123\":{\"pressure\":{\"output\":{\"magnitude\":0.270023,\"unit\":3},\"error\":{\"magnitude\":0.0086071311,\"unit\":7}},\"temperature\":{\"output\":{\"magnitude\":19.5347,\"unit\":4},\"error\":{\"magnitude\":-0.016222389,\"unit\":4}}}}}},{\"reference\":\"F_12300_XX_0000098765\",\"environmentTarget\":{\"pressure\":{\"magnitude\":0.35,\"unit\":3},\"temperature\":{\"magnitude\":20.0,\"unit\":4}},\"environment\":{\"pressure\":{\"magnitude\":0.350004,\"unit\":3},\"temperature\":{\"magnitude\":19.5509,\"unit\":4},\"supply\":{\"magnitude\":1.0,\"unit\":18}},\"raw\":{\"signal\":{\"magnitude\":59.992312915,\"unit\":22},\"bridgeResistance\":{\"magnitude\":3499.6249412,\"unit\":28}},\"compensated\":{\"mathematicalModels\":{\"MM0123\":{\"pressure\":{\"output\":{\"magnitude\":0.350004,\"unit\":3},\"error\":{\"magnitude\":0.00010743234,\"unit\":7}},\"temperature\":{\"output\":{\"magnitude\":19.5345,\"unit\":4},\"error\":{\"magnitude\":-0.01639968,\"unit\":4}}}}}},{\"reference\":\"F_12300_XX_0000098765\",\"environmentTarget\":{\"pressure\":{\"magnitude\":0.03,\"unit\":3},\"temperature\":{\"magnitude\":40.0,\"unit\":4}},\"environment\":{\"pressure\":{\"magnitude\":0.0300085,\"unit\":3},\"temperature\":{\"magnitude\":39.7284,\"unit\":4},\"supply\":{\"magnitude\":1.0,\"unit\":18}},\"raw\":{\"signal\":{\"magnitude\":17.397262944,\"unit\":22},\"bridgeResistance\":{\"magnitude\":3691.5753762,\"unit\":28}},\"compensated\":{\"mathematicalModels\":{\"MM0123\":{\"pressure\":{\"output\":{\"magnitude\":0.0300228,\"unit\":3},\"error\":{\"magnitude\":0.0040960795,\"unit\":7}},\"temperature\":{\"output\":{\"magnitude\":39.7199,\"unit\":4},\"error\":{\"magnitude\":-0.0085095008,\"unit\":4}}}}}},{\"reference\":\"F_12300_XX_0000098765\",\"environmentTarget\":{\"pressure\":{\"magnitude\":0.11,\"unit\":3},\"temperature\":{\"magnitude\":40.0,\"unit\":4}},\"environment\":{\"pressure\":{\"magnitude\":0.11,\"unit\":3},\"temperature\":{\"magnitude\":39.7284,\"unit\":4},\"supply\":{\"magnitude\":1.0,\"unit\":18}},\"raw\":{\"signal\":{\"magnitude\":28.371817632,\"unit\":22},\"bridgeResistance\":{\"magnitude\":3687.5127763,\"unit\":28}},\"compensated\":{\"mathematicalModels\":{\"MM0123\":{\"pressure\":{\"output\":{\"magnitude\":0.109974,\"unit\":3},\"error\":{\"magnitude\":-0.0074748965,\"unit\":7}},\"temperature\":{\"output\":{\"magnitude\":39.723,\"unit\":4},\"error\":{\"magnitude\":-0.0053894707,\"unit\":4}}}}}},{\"reference\":\"F_12300_XX_0000098765\",\"environmentTarget\":{\"pressure\":{\"magnitude\":0.19,\"unit\":3},\"temperature\":{\"magnitude\":40.0,\"unit\":4}},\"environment\":{\"pressure\":{\"magnitude\":0.190007,\"unit\":3},\"temperature\":{\"magnitude\":39.7284,\"unit\":4},\"supply\":{\"magnitude\":1.0,\"unit\":18}},\"raw\":{\"signal\":{\"magnitude\":39.328392738,\"unit\":22},\"bridgeResistance\":{\"magnitude\":3683.4440504,\"unit\":28}},\"compensated\":{\"mathematicalModels\":{\"MM0123\":{\"pressure\":{\"output\":{\"magnitude\":0.190006,\"unit\":3},\"error\":{\"magnitude\":-0.00034589005,\"unit\":7}},\"temperature\":{\"output\":{\"magnitude\":39.7184,\"unit\":4},\"error\":{\"magnitude\":-0.0099779654,\"unit\":4}}}}}},{\"reference\":\"F_12300_XX_0000098765\",\"environmentTarget\":{\"pressure\":{\"magnitude\":0.27,\"unit\":3},\"temperature\":{\"magnitude\":40.0,\"unit\":4}},\"environment\":{\"pressure\":{\"magnitude\":0.269992,\"unit\":3},\"temperature\":{\"magnitude\":39.7284,\"unit\":4},\"supply\":{\"magnitude\":1.0,\"unit\":18}},\"raw\":{\"signal\":{\"magnitude\":50.253005569,\"unit\":22},\"bridgeResistance\":{\"magnitude\":3679.4961501,\"unit\":28}},\"compensated\":{\"mathematicalModels\":{\"MM0123\":{\"pressure\":{\"output\":{\"magnitude\":0.270012,\"unit\":3},\"error\":{\"magnitude\":0.005662001,\"unit\":7}},\"temperature\":{\"output\":{\"magnitude\":39.7193,\"unit\":4},\"error\":{\"magnitude\":-0.0090714064,\"unit\":4}}}}}},{\"reference\":\"F_12300_XX_0000098765\",\"environmentTarget\":{\"pressure\":{\"magnitude\":0.35,\"unit\":3},\"temperature\":{\"magnitude\":40.0,\"unit\":4}},\"environment\":{\"pressure\":{\"magnitude\":0.349998,\"unit\":3},\"temperature\":{\"magnitude\":39.7284,\"unit\":4},\"supply\":{\"magnitude\":1.0,\"unit\":18}},\"raw\":{\"signal\":{\"magnitude\":61.143106082,\"unit\":22},\"bridgeResistance\":{\"magnitude\":3675.5825482,\"unit\":28}},\"compensated\":{\"mathematicalModels\":{\"MM0123\":{\"pressure\":{\"output\":{\"magnitude\":0.349977,\"unit\":3},\"error\":{\"magnitude\":-0.0059764458,\"unit\":7}},\"temperature\":{\"output\":{\"magnitude\":39.7162,\"unit\":4},\"error\":{\"magnitude\":-0.012197143,\"unit\":4}}}}}},{\"reference\":\"F_12300_XX_0000098765\",\"environmentTarget\":{\"pressure\":{\"magnitude\":0.03,\"unit\":3},\"temperature\":{\"magnitude\":60.0,\"unit\":4}},\"environment\":{\"pressure\":{\"magnitude\":0.0299943,\"unit\":3},\"temperature\":{\"magnitude\":59.8651,\"unit\":4},\"supply\":{\"magnitude\":1.0,\"unit\":18}},\"raw\":{\"signal\":{\"magnitude\":18.438349496,\"unit\":22},\"bridgeResistance\":{\"magnitude\":3894.7603133,\"unit\":28}},\"compensated\":{\"mathematicalModels\":{\"MM0123\":{\"pressure\":{\"output\":{\"magnitude\":0.0300107,\"unit\":3},\"error\":{\"magnitude\":0.0046958964,\"unit\":7}},\"temperature\":{\"output\":{\"magnitude\":59.9229,\"unit\":4},\"error\":{\"magnitude\":0.057798431,\"unit\":4}}}}}},{\"reference\":\"F_12300_XX_0000098765\",\"environmentTarget\":{\"pressure\":{\"magnitude\":0.11,\"unit\":3},\"temperature\":{\"magnitude\":60.0,\"unit\":4}},\"environment\":{\"pressure\":{\"magnitude\":0.110011,
